vi "shuttercontrol_multi.vi"(1 "error in":errorcluster, 2 "Autoshutter Chans":u32[](array[numeric]), 3 "command":string) -> (0 "error out":errorcluster)   [LabVIEW 2015]
uses:
  <vilib>/DAQmx/write.llb/DAQmx Write (Digital 1D Bool NChan 1Samp 1Line).vi
  <vilib>/DAQmx/create/channels.llb/DAQmx Create Channel (DO-Digital Output).vi
  <vilib>/DAQmx/miscellaneous.llb/DAQmx Fill In Error Info.vi
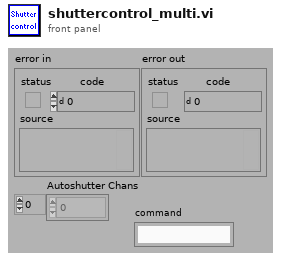
[diagram p1: front panel]
types:
  T1 = typedef "XYZStage.lvlib/XYZStage Configuration.ctl" = cluster{"VISA resource name":refnum<visa-resource-name>, "Timeout (3sec)":u32}
  T2 = cluster{"StageS":i32, "StageL":i32, "currmeas data dir":path, "image OD":u16, "contour OD":u16, "point OD":u16, "AOlines":tag[], "AIlines":tag[], "CI lines":tag[], "DO lines":tag[], "AO names":string[], "CI names":string[], "AI names":string[], "DO names":string[], "CIextensions":string[], "AIextensions":string[], "Voltage to Ygalvo":i32, "Voltage to Xgalvo":i32, "Voltage to patch":i32, "640 shutter":i32, "2P shutter":i32, "LT timestamp":u32, "Vp":i32, "Ip":i32, "camera trigger":i32, "master data dir":path, "voltage to Zpos":i32, "Vto2P":i32, "640 AO":i32, "488 AO":i32, "532 AO":i32, "640TTL":u32, "488TTL":u32, "532TTL":u32, "Device 1 sampleclock out":tag, "Device 1 Starttrigger out":tag, "Device 2 sampleclock in":tag, "Device 2 StartTrigger in ":tag, "2PODTTL":u32, "488 shutter":u32, "LCVR red":u32, "LCVR blue":u32, "Sutter Stage Config":T1, "Device 1 ext sampleclock in (100Khz)":tag}
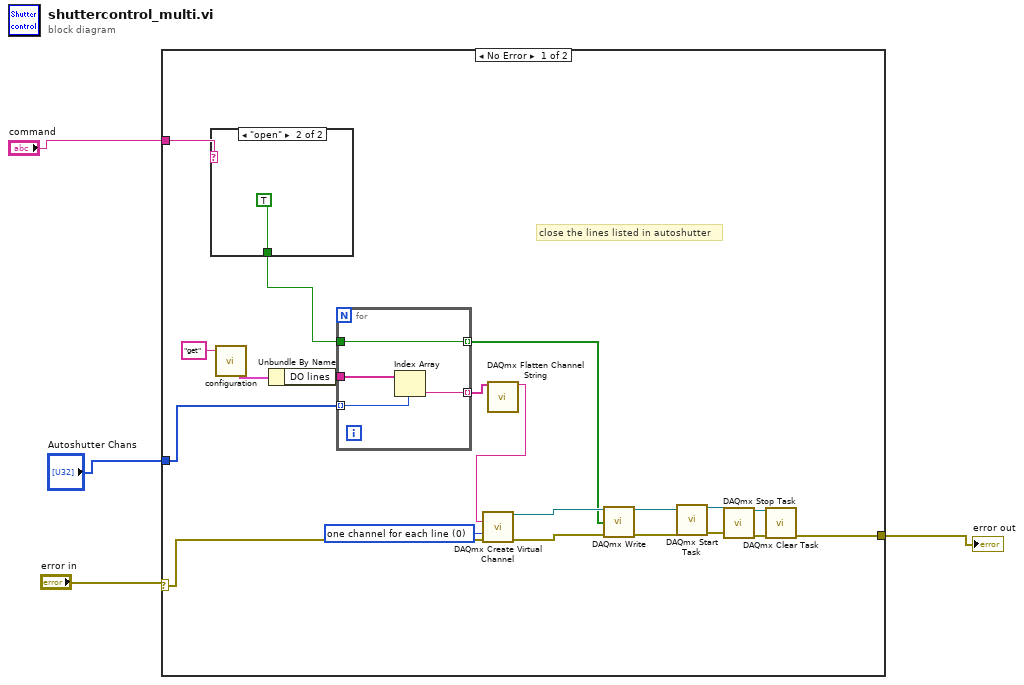
[diagram p0: block diagram]
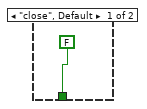
[diagram p2: hidden frame]
diagram:
  n1 = case shown="No Error" "error in" {
    selector: "error in" -> [w12 w31]
    tunnel: [w13 w31] -> w3
    tunnel: "command" -> [w11 _]
    tunnel: "Autoshutter Chans" -> [w10 _]
    frame No Error {
      w5 = 0 items=["one channel for each line", "one channel for all lines"] ("line grouping")
      # "close the lines listed in autoshutter"
      n2 = case shown="\"open\"" w11 {
        tunnel: [FALSE ("data") TRUE ("data")] -> w7
        frame "close", Default {
        }
        frame "open" {
        }
      }
      n3 = call "configuration.vi"("command"="get") -> ("config out"=w15:T2)  [unwired: 2 in, 1 out]
      n4 = Unbundle By Name(w15) -> ("DO lines"=w14:tag[])
      n5 = for {
        tunnel: w14 -> [w28]
        tunnel: w10 -> [w27] mode=indexing
        tunnel: [w26] -> w9 mode=indexing
        tunnel: w7 -> [w25]
        tunnel: [w25] -> w6 mode=indexing
        n6 = Index Array(array=w28, index=w27) -> (element=w26:tag)
      }
      n7 = call <vilib>:"DAQmx Flatten Channel String.vi"("names in"=w9) -> ("names out"=w8:string)  [unwired: 13 in, 1 out]
      n8 = call-poly <vilib>:"DAQmx Create Virtual Channel.vi"("lines"=w8, "line grouping"=w5, "error in"=w12) -> ("task out"=w18:refnum<k21>, "error out"=w17:errorcluster)  [unwired: 11 in]
      n9 = call-poly <vilib>:"DAQmx Write.vi"("task/channels in"=w18, "data"=w6, "error in"=w17) -> ("task out"=w19:refnum<k21>, "error out"=w20:errorcluster)  [unwired: 10 in, 1 out]
      n10 = call <vilib>:"DAQmx Start Task.vi"("task/channels in"=w19, "error in"=w20) -> ("task out"=w21:refnum<k21>, "error out"=w22:errorcluster)  [unwired: 12 in]
      n11 = call <vilib>:"DAQmx Stop Task.vi"("task/channels in"=w21, "error in"=w22) -> ("task out"=w23:refnum<k21>, "error out"=w24:errorcluster)  [unwired: 12 in]
      n12 = call <vilib>:"DAQmx Clear Task.vi"("task in"=w23, "error in"=w24) -> ("error out"=w13:errorcluster)  [unwired: 13 in]
    }
    frame Error {
    }
  }
  "error out" <- w3
